vi "Dequeue.vi"(8 "error in":errorcluster) -> (0 "error out":errorcluster, 2 "Data":variant, 3 "State":T1)   [LabVIEW 2018, in "Vehicle Position Interface.lvlib"]
uses:
  Vehicle Position Interface.lvlib
  ctl/Module State.ctl
  ctl/Queue Actions.ctl
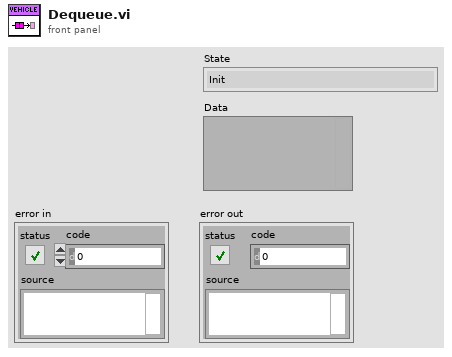
[diagram p1: front panel]
types:
  T1 = typedef "Vehicle Position Interface.lvlib/Module State.ctl" = enum16{"Init", "Idle", "Error", "Close", "Vehicle Position: Set", "Vehicle Position: Send to controller"}
  T2 = typedef "Vehicle Position Interface.lvlib/Queue Actions.ctl" = enum16{"Create", "Get", "Destroy"}
  T3 = typedef "Vehicle Position Interface.lvlib/Module Message.ctl" = cluster{"State":T1, "Data":variant}
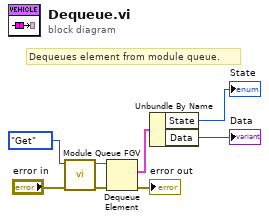
[diagram p0: block diagram]
diagram:
  # "Dequeues element from module queue."
  n1 = call "Module Queue FGV.vi"("error in"="error in", "Action"=Queue_Actions."Get") -> ("error out"=w2:errorcluster, "Queue ref"=w3:refnum<queue>)  [unwired: 8 in]
  n2 = Dequeue Element(queue=w3, error in (no error)=w2) -> (element=w6:T3, error out=→"error out":errorcluster)  [unwired: 1 in, 2 out]
  n3 = Unbundle By Name(w6) -> ("State"=→"State":T1, "Data"=→"Data":variant)
